vi "bufertest.vi"() -> ()   [LabVIEW 2010]
panel:
  in  "works/doesn't work":bool
  out "timeout 8":dbl
  out "timeout 7":dbl
  in  "timeout 6":dbl
  in  "timeout 5":dbl
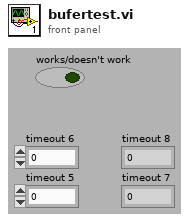
[diagram p1: front panel]
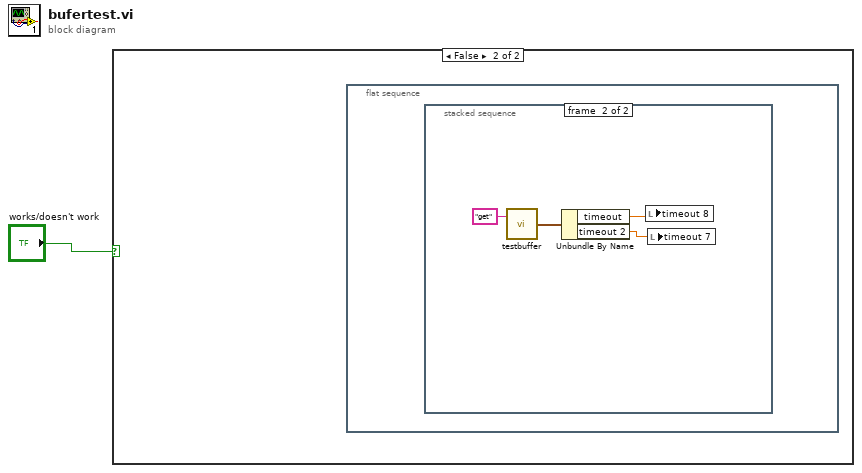
[diagram p0: block diagram]
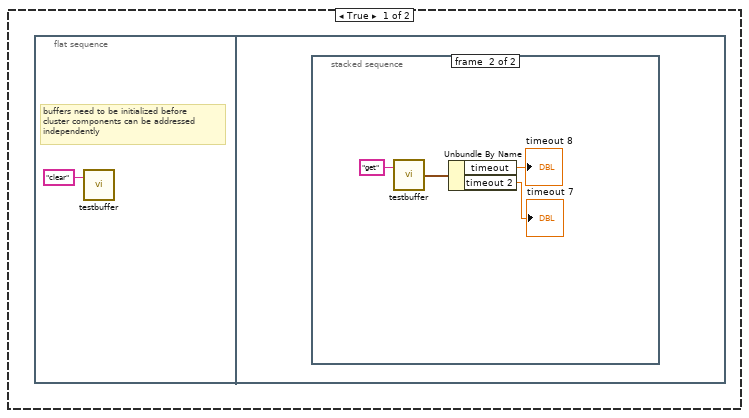
[diagram p2: hidden frame]
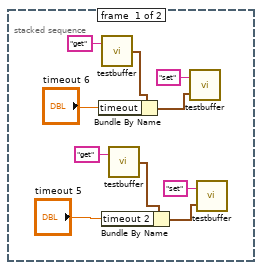
[diagram p3: hidden frame]
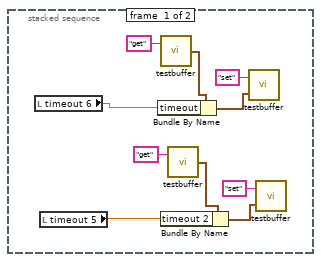
[diagram p4: hidden frame]
diagram:
  n1 = case shown="False" "works/doesn't work" {
    frame True {
      n2 = flat-sequence {
        frame #0 {
          # "buffers need to be initialized before\ncluster components can be addressed\nindependently"
          n3 = call "testbuffer.vi"("command"="clear") -> ()  [unwired: 1 in, 1 out]
        }
        frame #1 {
          n4 = stacked-sequence {
            frame #0 {
              n5 = call "testbuffer.vi"("command"="get") -> ("Temp Config out"=w10:cluster{"timeout":dbl, "timeout 2":dbl})  [unwired: 1 in]
              n6 = Bundle By Name(cluster=w10, "timeout"="timeout 6") -> (w9:cluster{"timeout":dbl, "timeout 2":dbl})
              n7 = call "testbuffer.vi"("command"="get") -> ("Temp Config out"=w6:cluster{"timeout":dbl, "timeout 2":dbl})  [unwired: 1 in]
              n8 = Bundle By Name(cluster=w6, "timeout 2"="timeout 5") -> (w7:cluster{"timeout":dbl, "timeout 2":dbl})
              n9 = call "testbuffer.vi"("Temp Config in"=w9, "command"="set") -> ()  [unwired: 1 out]
              n10 = call "testbuffer.vi"("Temp Config in"=w7, "command"="set") -> ()  [unwired: 1 out]
            }
            frame #1 {
              n11 = call "testbuffer.vi"("command"="get") -> ("Temp Config out"=w15:cluster{"timeout":dbl, "timeout 2":dbl})  [unwired: 1 in]
              n12 = Unbundle By Name(w15) -> ("timeout"=→"timeout 8":dbl, "timeout 2"=→"timeout 7":dbl)
            }
          }
        }
      }
    }
    frame False {
      n13 = flat-sequence {
        frame #0 {
          n14 = stacked-sequence {
            frame #0 {
              n15 = local read "timeout 6"() -> (w18:dbl)
              n16 = local read "timeout 5"() -> (w17:dbl)
              n17 = call "testbuffer.vi"("command"="get") -> ("Temp Config out"=w24:cluster{"timeout":dbl, "timeout 2":dbl})  [unwired: 1 in]
              n18 = Bundle By Name(cluster=w24, "timeout"=w18) -> (w23:cluster{"timeout":dbl, "timeout 2":dbl})
              n19 = call "testbuffer.vi"("command"="get") -> ("Temp Config out"=w21:cluster{"timeout":dbl, "timeout 2":dbl})  [unwired: 1 in]
              n20 = Bundle By Name(cluster=w21, "timeout 2"=w17) -> (w22:cluster{"timeout":dbl, "timeout 2":dbl})
              n21 = call "testbuffer.vi"("Temp Config in"=w23, "command"="set") -> ()  [unwired: 1 out]
              n22 = call "testbuffer.vi"("Temp Config in"=w22, "command"="set") -> ()  [unwired: 1 out]
            }
            frame #1 {
              n23 = call "testbuffer.vi"("command"="get") -> ("Temp Config out"=w29:cluster{"timeout":dbl, "timeout 2":dbl})  [unwired: 1 in]
              n24 = Unbundle By Name(w29) -> ("timeout"=w28:dbl, "timeout 2"=w27:dbl)
              n25 = local write "timeout 8"(w28) -> ()
              n26 = local write "timeout 7"(w27) -> ()
            }
          }
        }
      }
    }
  }
